vi "fp5ultra.vi"   [LabVIEW 2016]
uses:
  <vilib>/NXT/Block Support/NXT_OutputPort.ctl
  <vilib>/NXT/Block Support/NXT_InputPort.ctl
  <vilib>/NXT/NXTIO Xnodes/NXTIONodeSubVIs/LEGOResetMotors.vi
  <vilib>/NXT/Dual Mode Library/Sensors/EV3_Ultrasonic_CM.vi
  <vilib>/NXT/Dual Mode Library/Sensors/EV3_Color_Reflect.vi
  <vilib>/NXT/NXTIO Xnodes/NXTIONodeSubVIs/NXTMoveMotors.vi
  <vilib>/NXT/NXTIO Xnodes/NXTIONodeSubVIs/NXTMotorRunDistance.vi
  <vilib>/NXT/NXTIO Xnodes/NXTIONodeSubVIs/NXTStopMotors.vi
  <vilib>/NXT/Dual Mode Library/Sound/PlayAsharp.vi
  <vilib>/NXT/Dual Mode Library/Sound/PlayC.vi
  <vilib>/NXT/Subs/LVHSConnector.ctl
  <vilib>/NXT/NXTIO Xnodes/AddressXNode/NXTIOAddress.xnode
  <vilib>/NXT/NXTIO Xnodes/NXTIOXNode/NXTIO.xnode
  <vilib>/NXT/LegoClasses/BrickReference/BrickReference.lvclass
types:
  T1 = typedef "NXT_OutputPort.ctl" = u8
  T2 = typedef "NXT_InputPort.ctl" = u32
  T3 = typedef "LVHSConnector.ctl" = refnum<class "BrickReference.lvclass">
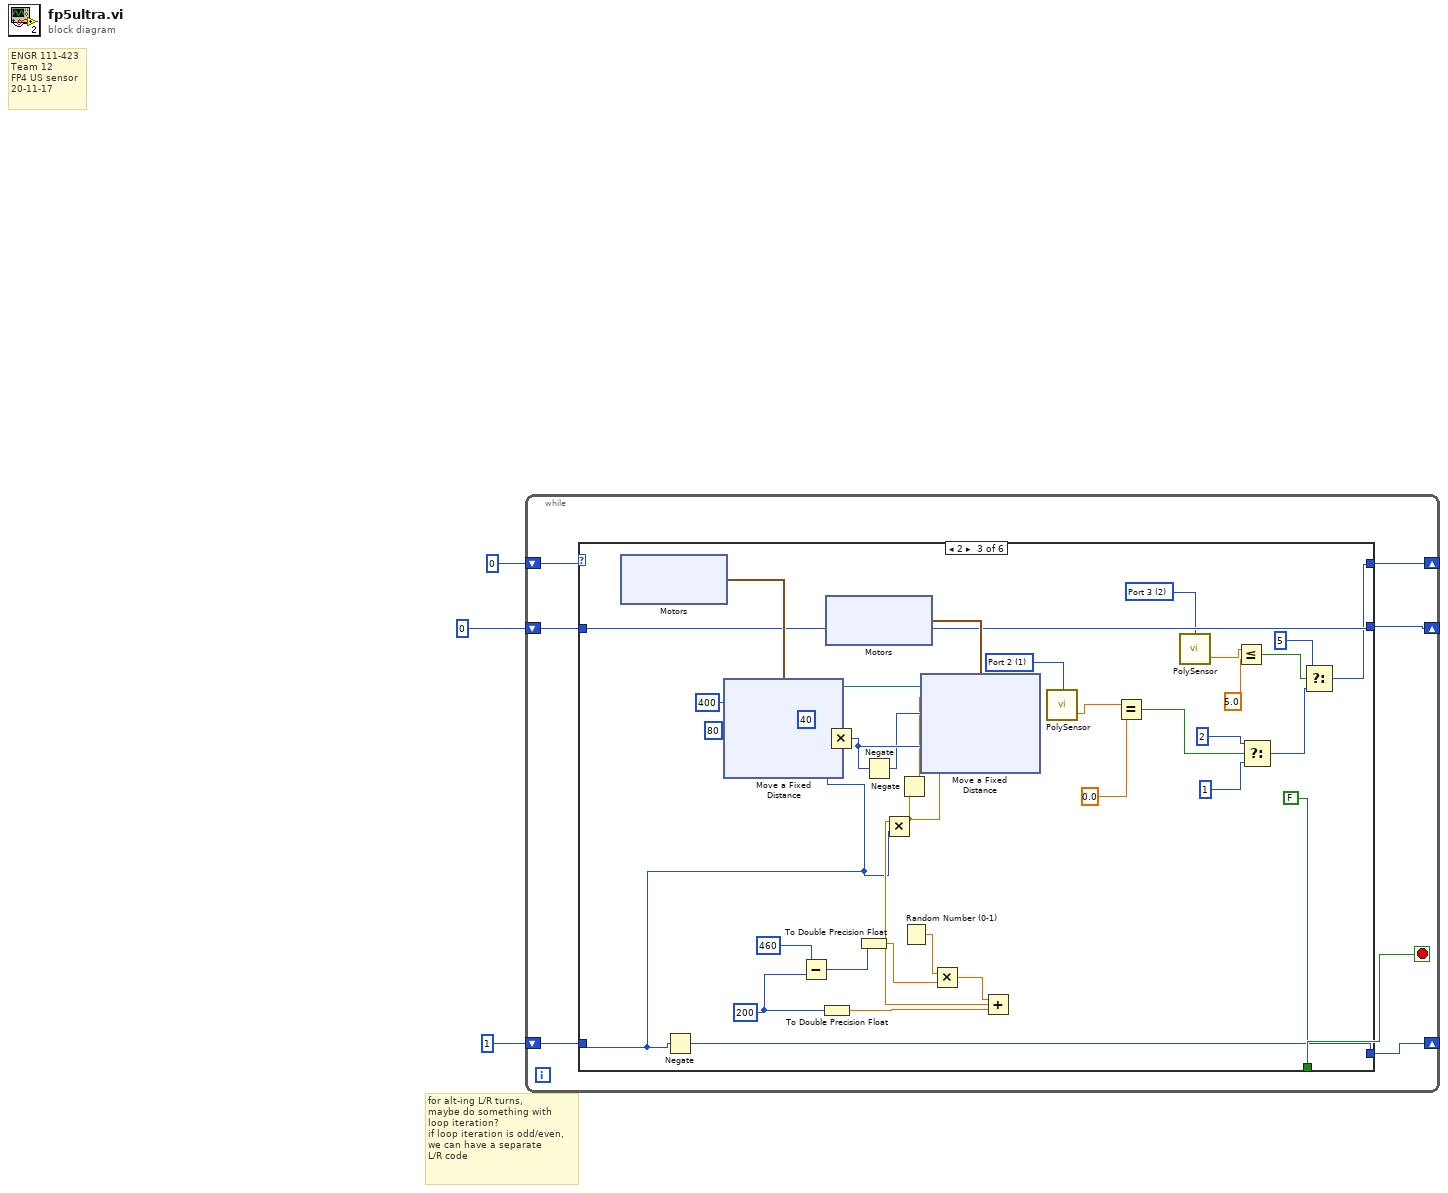
[diagram p0: block diagram]
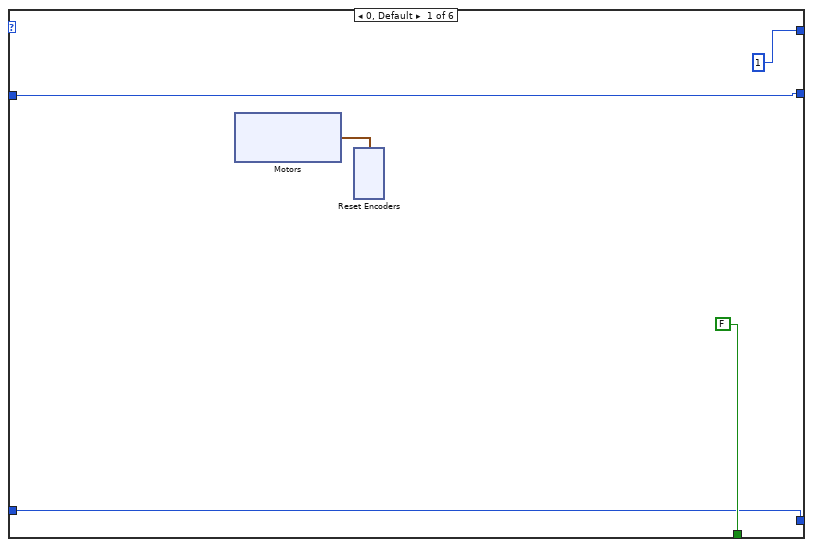
[diagram p2: hidden frame]
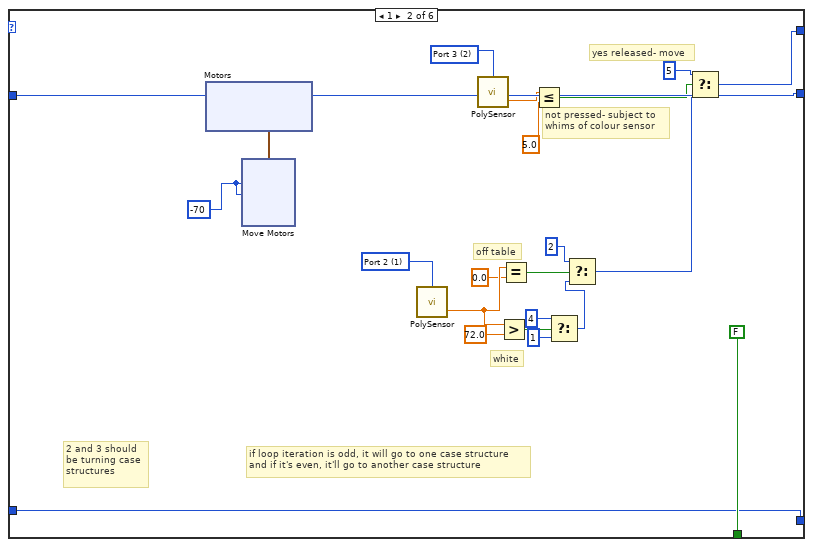
[diagram p3: hidden frame]
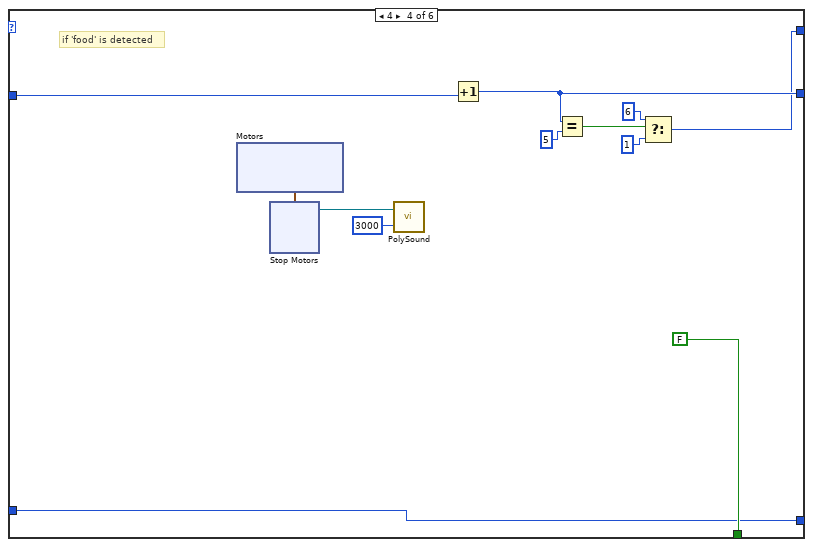
[diagram p4: hidden frame]
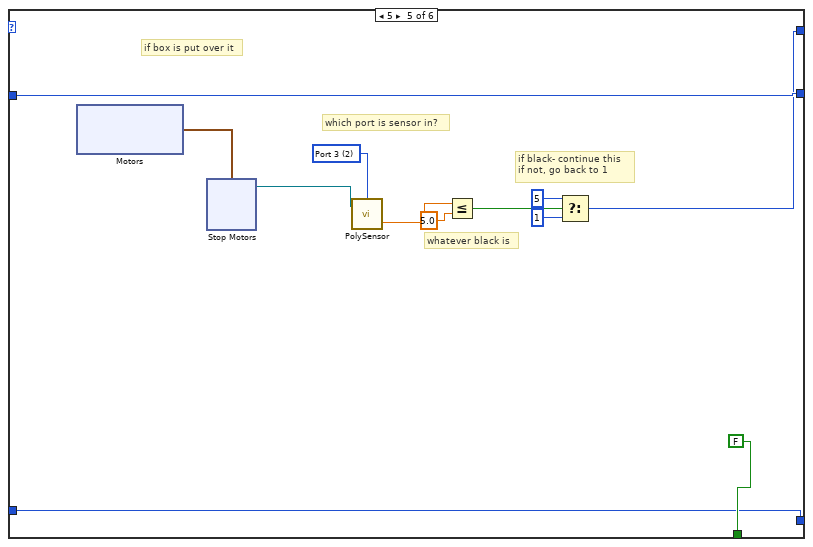
[diagram p5: hidden frame]
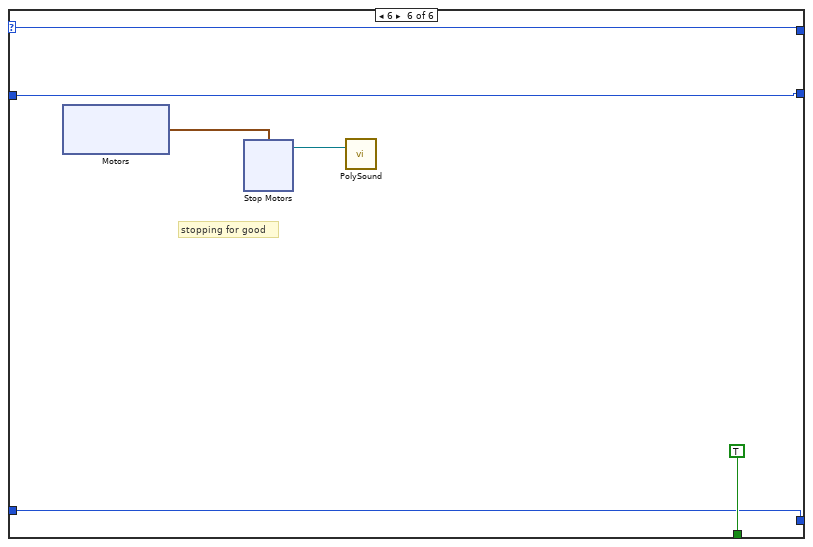
[diagram p6: hidden frame]
diagram:
  # "for alt-ing L/R turns,\nmaybe do something with\nloop iteration?\nif loop iteration is odd/even,\nwe can have a separate\nL/R code"
  # "ENGR 111-423\nTeam 12\nFP4 US sensor\n20-11-17"
  n1 = while {
    shift-right: [w8] -> _
    shift-left: 0 -> [w10]
    shift-right: [w6] -> _
    shift-left: 0 -> [w7]
    shift-right: [w4] -> _
    shift-left: 1 -> [w5]
    stop <- w9 stop-if-true
    n2 = case shown="2" w10 {
      selector: w10 -> [_ _ _ _ _ w155]
      tunnel: [FALSE FALSE FALSE FALSE FALSE TRUE] -> w9
      tunnel: [1 w33 w68 w116 w138 w155] -> w8
      tunnel: w7 -> [w12 w29 w69 w123 w140 w152]
      tunnel: [w12 w29 w69 w120 w140 w152] -> w6
      tunnel: w5 -> [w11 w25 w52 w115 w139 w151]
      tunnel: [w11 w25 w53 w115 w139 w151] -> w4
      frame 0, Default {
        n3 = xnode "Motors"() -> ("Motor"=w13:cluster{"Port":T1, "Port":T1})
        n4 = xnode "Reset Encoders"("Motors"=w13) -> ()  [unwired: 1 in, 1 out]
      }
      frame 1 {
        w34 = T2 1 items=["Port 1", "Port 2", "Port 3", "Port 4"] ("Port (Port 1)")
        w21 = T2 2 items=["Port 1", "Port 2", "Port 3", "Port 4"] ("Port (Port 1)")
        w41 = -70 ("Distance 1")
        # "white"
        # "off table"
        # "2 and 3 should\nbe turning case\nstructures"
        # "if loop iteration is odd, it will go to one case structure\nand if it's even, it'll go to another case structure"
        # "not pressed- subject to\nwhims of colour sensor"
        # "yes released- move"
        n5 = xnode "Motors"() -> ("Motor"=w42:cluster{"Port":T1, "Port":T1})
        n6 = xnode "Move Motors"("Power/Speed 2"=w41, "Power/Speed 1"=w41, "Motors"=w42) -> ()  [unwired: 1 in, 1 out]
        n7 = call-poly <vilib>:"PolySensor.vi"("Port (Port 1)"=w34) -> ("Scaled Value"=w35:sgl)  [unwired: 2 in, 1 out]
        n8 = call-poly <vilib>:"PolySensor.vi"("Port (Port 1)"=w21) -> ("Centimeters"=w24:sgl)  [unwired: 2 in, 1 out]
        n9 = Greater?(x=w35, y=sgl 72.0) -> (0:w39:bool)
        n10 = Equal?(x=w35, y=sgl 0.0) -> (x = y?=w37:bool)
        n11 = Less Or Equal?(x=w24, y=sgl 5.0) -> (x <= y?=w22:bool)
        n12 = Select(t=i16 4, s=w39, f=i16 1) -> (s? t:f=w31:i16)
        n13 = Select(t=2, s=w37, f=w31) -> (s? t:f=w26:i32)
        n14 = Select(t=i16 5, s=w22, f=w26) -> (s? t:f=w33:i32)
      }
      frame 2 {
        w65 = 200
        w76 = 80 ("Distance 1")
        w77 = 400 ("Distance 1")
        w81 = T2 1 items=["Port 1", "Port 2", "Port 3", "Port 4"] ("Port (Port 1)")
        w57 = T2 2 items=["Port 1", "Port 2", "Port 3", "Port 4"] ("Port (Port 1)")
        n15 = xnode "Motors"() -> ("Motor"=w78:cluster{"Port":T1, "Port":T1})
        n16 = Negate(x=w52) -> (-x=w53:i32)
        n17 = xnode "Move a Fixed Distance"("Speed 2"=w76, "Speed 1"=w76, "Distance 2"=w77, "Distance 1"=w77, "Motors"=w78) -> ("NXT/EV3"=w58:T3)  [unwired: 2 in]
        n18 = Subtract(x=460, y=w65) -> (x-y=w66:i32)
        n19 = To Double Precision Float(number=w65) -> (double precision float=w61:dbl)
        n20 = xnode "Motors"() -> ("Motor"=w79:cluster{"Port":T1, "Port":T1})
        n21 = Multiply(x=40 ("Distance 1"), y=w52) -> (x*y=w73:i32)
        n22 = To Double Precision Float(number=w66) -> (double precision float=w64:dbl)
        n23 = Negate(x=w73) -> (-x=w72:i32)
        n24 = Random Number (0-1)() -> (number: 0 to 1=w63:dbl)
        n25 = Multiply(x=w63, y=w64) -> (x*y=w62:dbl)
        n26 = Add(x=w62, y=w61) -> (x+y=w60:dbl)
        n27 = Multiply(x=w60, y=w52) -> (x*y=w59:dbl)
        n28 = Negate(x=w59) -> (-x=w71:dbl)
        n29 = xnode "Move a Fixed Distance"("Speed 2"=w73, "Speed 1"=w72, "Distance 2"=w59, "Distance 1"=w71, "Motors"=w79, "NXT/EV3"=w58) -> ()  [unwired: 1 in, 1 out]
        n30 = call-poly <vilib>:"PolySensor.vi"("Port (Port 1)"=w81) -> ("Scaled Value"=w80:sgl)  [unwired: 2 in, 1 out]
        n31 = Equal?(x=w80, y=0.0) -> (x = y?=w82:bool)
        n32 = call-poly <vilib>:"PolySensor.vi"("Port (Port 1)"=w57) -> ("Centimeters"=w56:sgl)  [unwired: 2 in, 1 out]
        n33 = Less Or Equal?(x=w56, y=sgl 5.0) -> (x <= y?=w54:bool)
        n34 = Select(t=2, s=w82, f=1) -> (s? t:f=w85:i32)
        n35 = Select(t=5, s=w54, f=w85) -> (s? t:f=w68:i32)
      }
      frame 4 {
        # "if 'food' is detected"
        n36 = xnode "Motors"() -> ("Motor"=w125:cluster{"Port":T1, "Port":T1})
        n37 = xnode "Stop Motors"("Motors"=w125) -> ("NXT/EV3"=w126:T3)  [unwired: 1 in]
        n38 = call-poly <vilib>:"PolySound.vi"("Duration (500 ms)"=u16 3000, "NXT/EV3"=w126) -> ()  [unwired: 2 in, 1 out]
        n39 = Increment(x=w123) -> (x+1=w120:i32)
        n40 = Equal?(x=w120, y=5) -> (x = y?=w121:bool)
        n41 = Select(t=6, s=w121, f=1) -> (s? t:f=w116:i32)
      }
      frame 5 {
        w136 = T2 2 items=["Port 1", "Port 2", "Port 3", "Port 4"] ("Port (Port 1)")
        # "if black- continue this\nif not, go back to 1"
        # "whatever black is"
        # "which port is sensor in?"
        # "if box is put over it"
        n42 = xnode "Motors"() -> ("Motor"=w144:cluster{"Port":T1, "Port":T1})
        n43 = xnode "Stop Motors"("Motors"=w144) -> ("NXT/EV3"=w137:T3)  [unwired: 1 in]
        n44 = call-poly <vilib>:"PolySensor.vi"("NXT/EV3"=w137, "Port (Port 1)"=w136) -> ("Centimeters"=w135:sgl)  [unwired: 1 in, 1 out]
        n45 = Less Or Equal?(x=w135, y=sgl 5.0) -> (x <= y?=w133:bool)
        n46 = Select(t=i16 5, s=w133, f=i16 1) -> (s? t:f=w138:i16)
      }
      frame 6 {
        # "stopping for good"
        n47 = xnode "Motors"() -> ("Motor"=w156:cluster{"Port":T1, "Port":T1})
        n48 = xnode "Stop Motors"("Motors"=w156) -> ("NXT/EV3"=w153:T3)  [unwired: 1 in]
        n49 = call-poly <vilib>:"PolySound.vi"("NXT/EV3"=w153) -> ()  [unwired: 3 in, 1 out]
      }
    }
  }
